vi "Init.vi"(8 "error in (no error)":errorcluster, 11 "DtoA in":refnum<class "No Clock.lvclass">) -> (0 "error out":errorcluster, 3 "DtoA out":refnum<class "No Clock.lvclass">)   [LabVIEW 2015, in "No Clock.lvclass"]
uses:
  No Clock.lvclass
  External Clock.lvclass
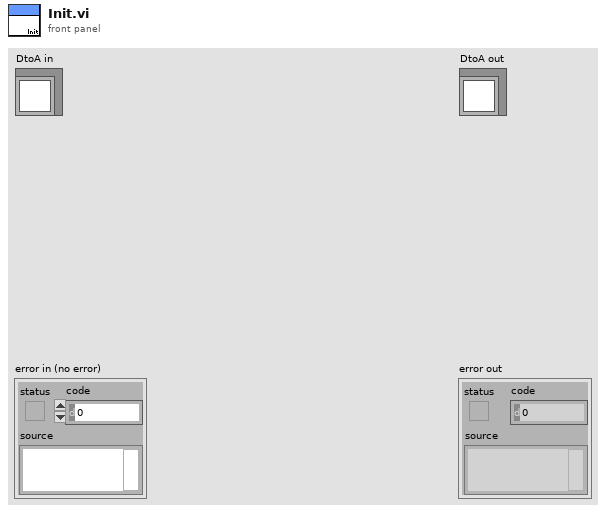
[diagram p1: front panel]
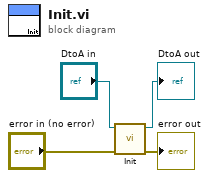
[diagram p0: block diagram]
diagram:
  n1 = call-parent "Init.vi"("error in (no error)"="error in (no error)", "DtoA in"="DtoA in") -> ("error out"=→"error out":errorcluster, "DtoA out"=→"DtoA out":refnum<class "No Clock.lvclass">)  [unwired: 8 in]
